vi "Test Copy from Pixmap ARGB.vi"(8 "error in (no error)":errorcluster, 11 "Test Case In":refnum<class "Image.lvclass">) -> (0 "error out":errorcluster, 3 "Test Case Out":refnum<class "Image.lvclass">)   [LabVIEW 2020, in "test.lvlib" / "Image.lvclass"]
uses:
  Image.lvclass
  C:/Program Files (x86)/National Instruments/LabVIEW 2020/vi.lib/Astemes/LUnit/Test Case.lvclass
  <vilib>/picture/picture.llb/imagedata.ctl
  <vilib>/Astemes/LUnit/Test Case.lvclass/Test Case.ctl
  2c93f62b-78d7-4b59-b27c-14bd701a5d71.vi
  26ba0610-68e5-456e-b31e-3dd4b1a41919.vi
  50a666bd-4679-4783-837b-c667b5268c61.vi
  5112621f-71fb-42da-a54b-011c251ba454.vi
  935961b4-3727-4f5b-bf0e-a61aebcf0dca.vi
  image/New Image (ARGB).vi
  image/New Image (Greyscale).vi
  image/Copy Pixmap to Image (ARGB with Mask Output).vi
  image/Copy Pixmap to Image (ARGB Flatten Mask).vi
  7f5bb767-9dbf-47d9-8f44-5f4901e96d00.vi
  e6d5ae8e-bd70-4c65-a769-b7cfb03e80c7.vi
  d454bffa-6717-48ab-b8d5-b1f03345aa55.vi
  image/New Image (ARGB).vi/3321fa97-f432-4e1e-8db9-a0df79aed21b.vi
  image/ARGB Colour to U32 Pixel Value.vi
  image/New Image (Greyscale).vi/6598b9e0-8a08-46f5-91fd-ca1b87217137.vi
  image/Copy Pixmap to Image (ARGB with Mask Output).vi/a116197e-b340-4968-94fb-08de404a21d3.vi
  image/Copy Pixmap to Image (ARGB Flatten Mask).vi/7d03ccf7-b889-4e8d-9f2a-57831e73dbde.vi
  <vilib>/Astemes/LUnit/Append Pass Result.vi
  <vilib>/Astemes/LUnit/Append Fail Result.vi
  <vilib>/Astemes/LUnit/Describe Comparison.vi
  7f5bb767-9dbf-47d9-8f44-5f4901e96d00.vi/9c5d11cd-9439-4240-a1ee-d9baace9c924.vi
  e6d5ae8e-bd70-4c65-a769-b7cfb03e80c7.vi/9c5d11cd-9439-4240-a1ee-d9baace9c924.vi
  d454bffa-6717-48ab-b8d5-b1f03345aa55.vi/9c5d11cd-9439-4240-a1ee-d9baace9c924.vi
  image/FixPixmap.vi
  <vilib>/Astemes/LUnit/Run In UI.vi
  image/Default8bitColourMap.vi
  <vilib>/Utility/error.llb/Clear Errors.vi
  common/Module Path.vi
  <vilib>/Utility/error.llb/Error Cluster From Error Code.vi
  <vilib>/Astemes/LUnit/Describe Variant.vi
  image/image.lvlib
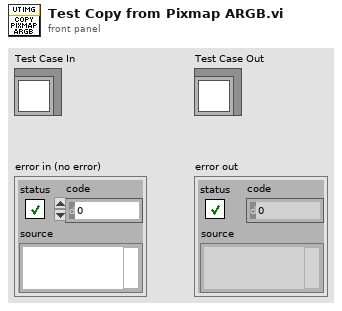
[diagram p1: front panel]
types:
  T1 = enum16{"8 Bit No Mask", "24 Bit No Mask", "32 Bit No Mask", "8 Bit Mask", "24 Bit Mask", "32 Bit Mask", "8 Pixels Wide Masked", "16 Pixels Wide Masked", "8 Bit No Colour Map"}
  T2 = cluster{"left":i16, "top":i16, "right":i16, "bottom":i16}
  T3 = enum16{"8 Bit No Mask", "24 Bit No Mask", "32 Bit No Mask", "8 Bit Mask", "24 Bit Mask", "32 Bit Mask", "8 Pixels Wide Masked", "16 Pixels Wide Masked", "8 Bit No Colour Map"}[]
  T4 = typedef "imagedata.ctl" = cluster{"image type":i32, "image depth":i32, "image":u8[], "mask":u8[], "colors":u32[], "Rectangle":cluster{"left":i16, "top":i16, "right":i16, "bottom":i16}}
  T5 = cluster{"8 No Mask":T4, "8 Mask":T4, "24 No Mask":T4, "24 Mask":T4, "32 No Mask":T4, "32 Mask":T4, "24 Mask - 8 wide":T4, "24 Mask - 16 wide":T4, "8 Bit No Colour Map":T4}
  T6 = typedef "image.lvlib/ARGB Image.ctl" = refnum<data-value>
  T7 = typedef "image.lvlib/Greyscale Image.ctl" = refnum<data-value>
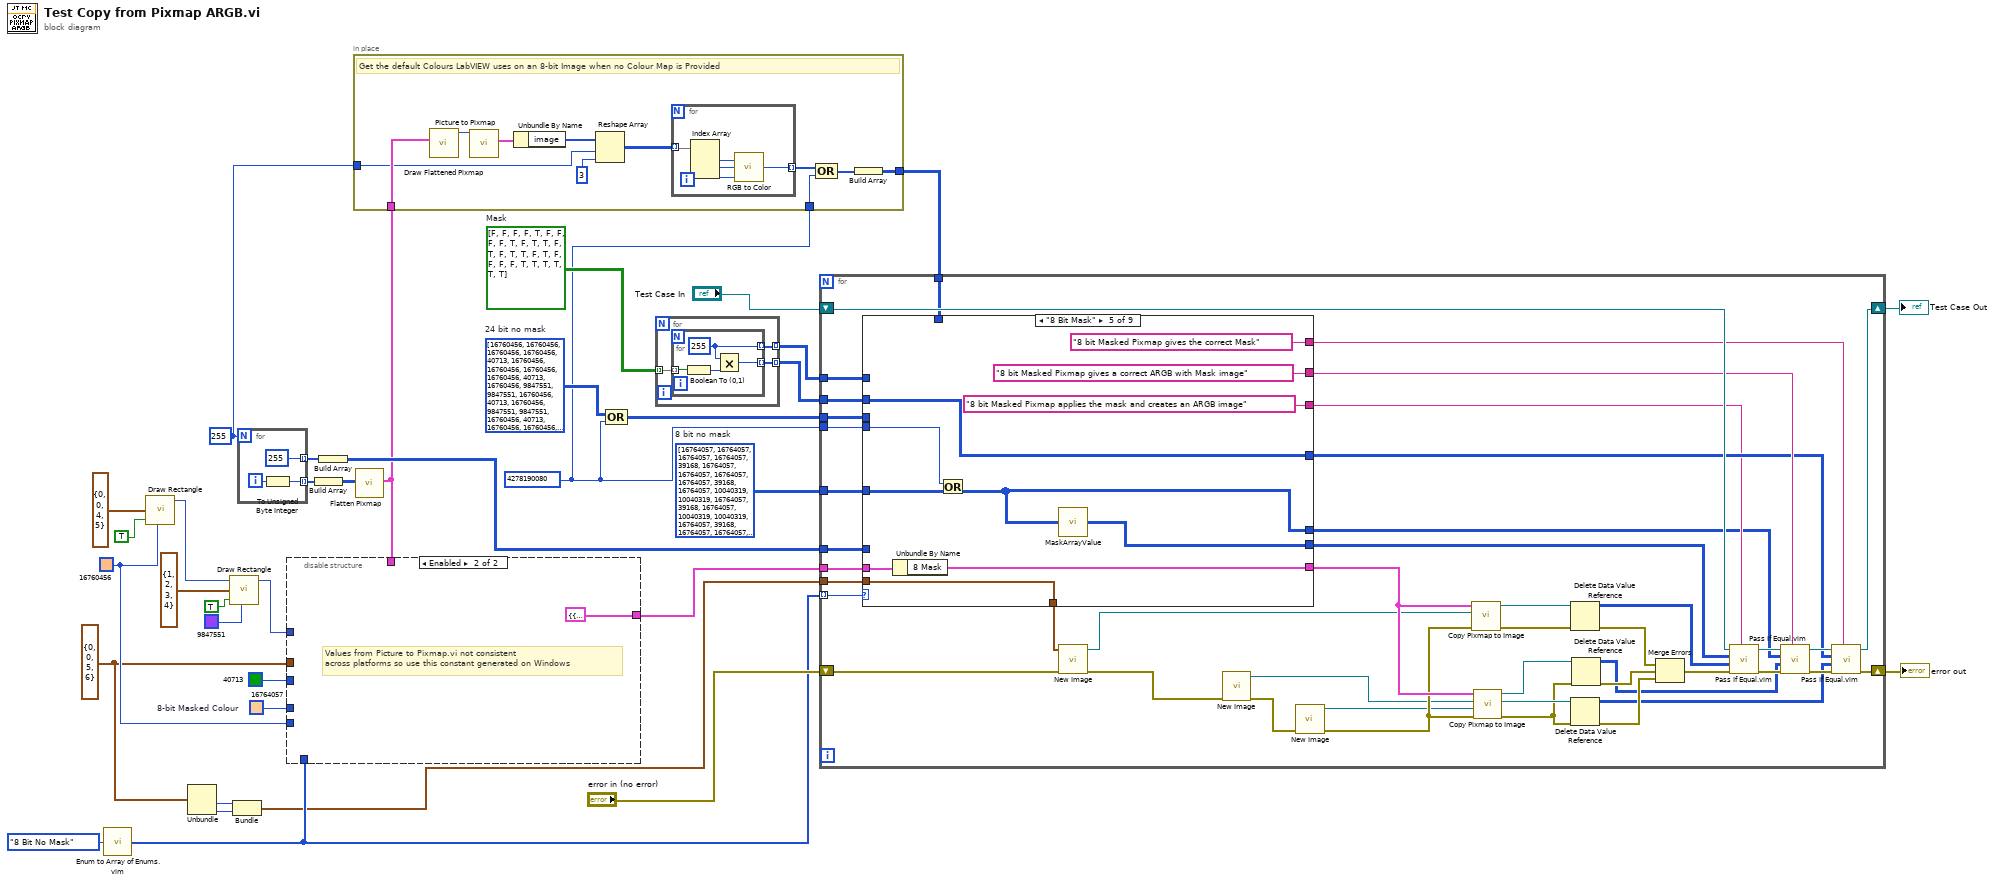
[diagram p0: block diagram]
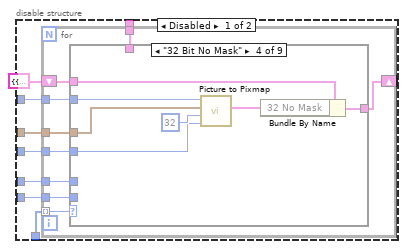
[diagram p2: hidden frame]
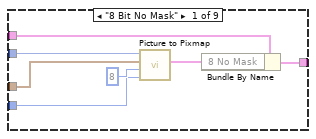
[diagram p3: hidden frame]
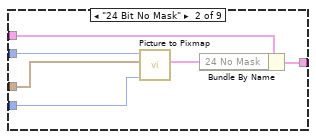
[diagram p4: hidden frame]
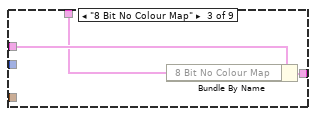
[diagram p5: hidden frame]
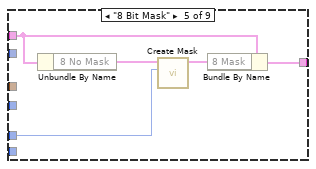
[diagram p6: hidden frame]
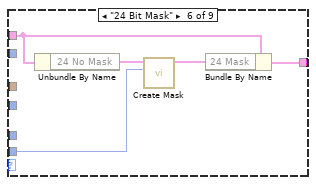
[diagram p7: hidden frame]
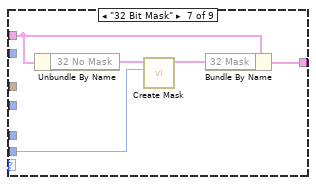
[diagram p8: hidden frame]
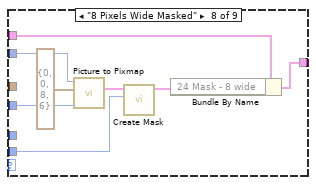
[diagram p9: hidden frame]
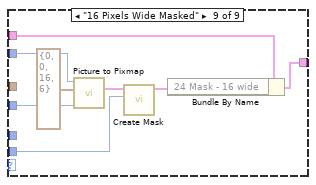
[diagram p10: hidden frame]
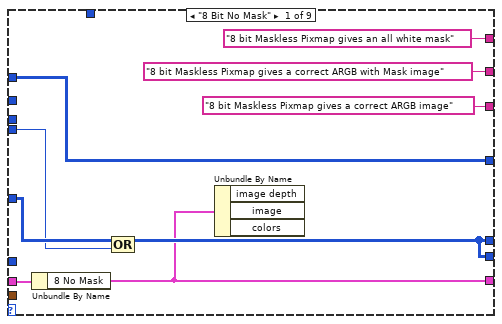
[diagram p11: hidden frame]
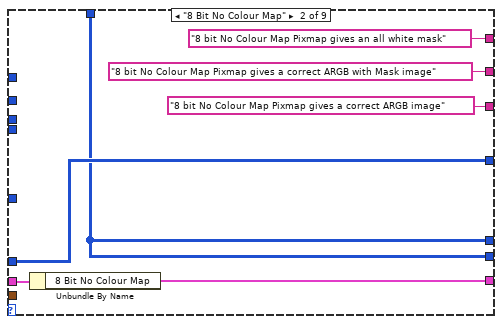
[diagram p12: hidden frame]
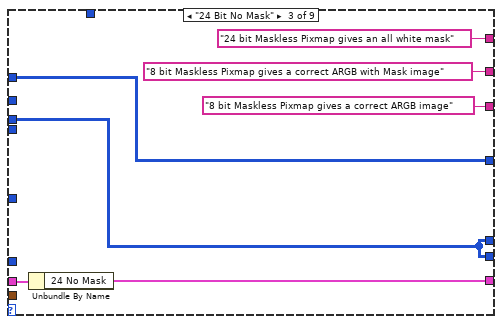
[diagram p13: hidden frame]
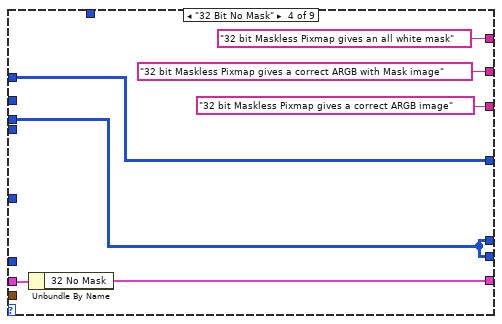
[diagram p14: hidden frame]
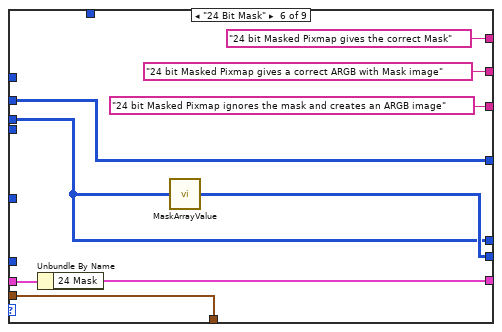
[diagram p15: hidden frame]
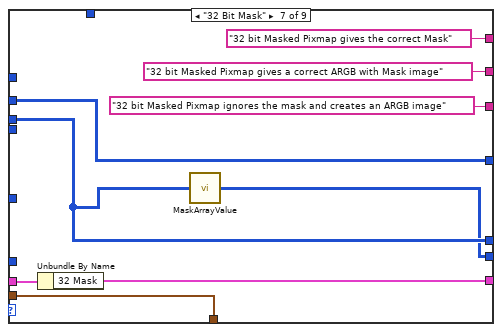
[diagram p16: hidden frame]
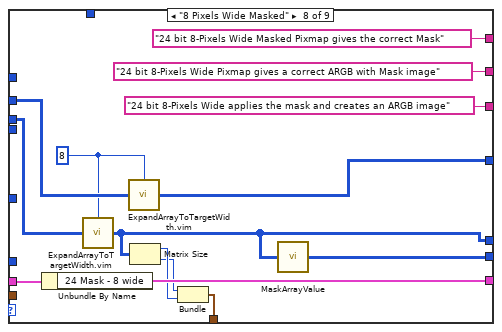
[diagram p17: hidden frame]
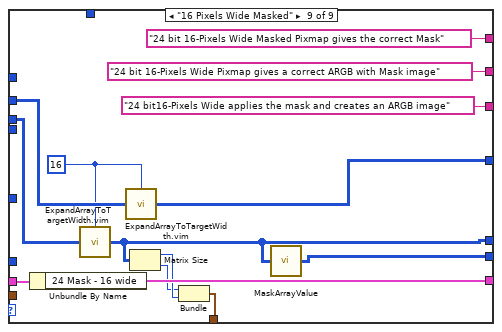
[diagram p18: hidden frame]
diagram:
  w1 = 255
  w9 = u32 16764057  # 8-bit Masked Colour
  w22 = bool[][] [[FALSE, FALSE, FALSE, FALSE, TRUE], [FALSE, FALSE, FALSE, FALSE, TRUE], [FALSE, TRUE, TRUE, FALSE, TRUE], [FALSE, TRUE, TRUE, FALSE, TRUE], [FALSE, FALSE, FALSE, FALSE, TRUE], [TRUE, TRUE, TRUE, TRUE, TRUE]]  # Mask
  w10 = u32[][] [[16764057, 16764057, 16764057, 16764057, 39168], [16764057, 16764057, 16764057, 16764057, 39168], [16764057, 10040319, 10040319, 16764057, 39168], [16764057, 10040319, 10040319, 16764057, 39168], [16764057, 16764057, 16764057, 16764057, 39168], [39168, 39168, 39168, 39168, 39168]]  # 8 bit no mask
  w2 = u32 4278190080
  w25 = u32[][] [[16760456, 16760456, 16760456, 16760456, 40713], [16760456, 16760456, 16760456, 16760456, 40713], [16760456, 9847551, 9847551, 16760456, 40713], [16760456, 9847551, 9847551, 16760456, 40713], [16760456, 16760456, 16760456, 16760456, 40713], [40713, 40713, 40713, 40713, 40713]]  # 24 bit no mask
  w14 = T2 {"left"=0, "top"=0, "right"=5, "bottom"=6} ("rect")
  w17 = u32 16760456 ("color(black)")
  n1 = call "Enum to Array of Enums.vim"("enum"=T1."8 Bit No Mask") -> ("array of enums"=w20:T3)
  n2 = call <vilib>:"Draw Rectangle.vi"("rect"=T2 {"left"=0, "top"=0, "right"=4, "bottom"=5}, "fill?(F)"=TRUE, "color(black)"=w17) -> ("new picture"=w35:picture)  [unwired: 6 in]
  n3 = Unbundle(w14) -> ("right"=w13:i16, "bottom"=w12:i16)  [unwired: 2 out]
  n4 = call <vilib>:"Draw Rectangle.vi"("picture"=w35, "rect"=T2 {"left"=1, "top"=2, "right"=3, "bottom"=4}, "fill?(F)"=TRUE, "color(black)"=u32 9847551) -> ("new picture"=w18:picture)  [unwired: 5 in]
  n5 = Bundle("right"=w13, "bottom"=w12) -> (w11:cluster{"right":i16, "bottom":i16})  [unwired: 1 in]
  n6 = for {
    N: w1 -> [_]
    tunnel: [w37] -> w8 mode=indexing
    tunnel: [u8 255 ("unsigned 8bit integer")] -> w6 mode=indexing
    i -> [w38]
    n7 = To Unsigned Byte Integer(number=w38) -> (unsigned 8bit integer=w37:u8)
  }
  n8 = Build Array(w8) -> (w7:u8[][])
  n9 = Build Array(w6) -> (w5:u8[][])
  n10 = call <vilib>:"Flatten Pixmap.vi"("8-bit pixmap"=w7) -> ("image data"=w4:T4)  [unwired: 10 in]
  n11 = disable-structure shown="Enabled" {
    disable-tunnel: w20 -> [w47 _]
    disable-tunnel: [w45 T5 {"8 No Mask"={"image type"=0, "image depth"=8, "image"=[8, 8, 8, 8, 197, 0, 8, 8, 8, 8, 197, 0, 8, 96, 96, 8, 197, 0, 8, 96, 96, 8, 197, 0, 8, 8, 8, 8, 197, 0, 197, 197, 197, 197, 197, 0], "mask"=[], "colors"=[16777215, 16777164, 16777113, 16777062, 16777011, 16776960, 16764159, 16764108, 16764057, 16764006, 16763955, 16763904, 16751103, 16751052, 16751001, 16750950, 16750899, 16750848, 16738047, 16737996, 16737945, 16737894, 16737843, 16737792, 16724991, 16724940, 16724889, 16724838, 16724787, 16724736, 16711935, 16711884, 16711833, 16711782, 16711731, 16711680, 13434879, 13434828, 13434777, 13434726, 13434675, 13434624, 13421823, 13421772, 13421721, 13421670, 13421619, 13421568, 13408767, 13408716, 13408665, 13408614, 13408563, 13408512, 13395711, 13395660, 13395609, 13395558, 13395507, 13395456, 13382655, 13382604, 13382553, 13382502, 13382451, 13382400, 13369599, 13369548, 13369497, 13369446, 13369395, 13369344, 10092543, 10092492, 10092441, 10092390, 10092339, 10092288, 10079487, 10079436, 10079385, 10079334, 10079283, 10079232, 10066431, 10066380, 10066329, 10066278, 10066227, 10066176, 10053375, 10053324, 10053273, 10053222, 10053171, 10053120, 10040319, 10040268, 10040217, 10040166, 10040115, 10040064, 10027263, 10027212, 10027161, 10027110, 10027059, 10027008, 6750207, 6750156, 6750105, 6750054, 6750003, 6749952, 6737151, 6737100, 6737049, 6736998, 6736947, 6736896, 6724095, 6724044, 6723993, 6723942, 6723891, 6723840, 6711039, 6710988, 6710937, 6710886, 6710835, 6710784, 6697983, 6697932, 6697881, 6697830, 6697779, 6697728, 6684927, 6684876, 6684825, 6684774, 6684723, 6684672, 3407871, 3407820, 3407769, 3407718, 3407667, 3407616, 3394815, 3394764, 3394713, 3394662, 3394611, 3394560, 3381759, 3381708, 3381657, 3381606, 3381555, 3381504, 3368703, 3368652, 3368601, 3368550, 3368499, 3368448, 3355647, 3355596, 3355545, 3355494, 3355443, 3355392, 3342591, 3342540, 3342489, 3342438, 3342387, 3342336, 65535, 65484, 65433, 65382, 65331, 65280, 52479, 52428, 52377, 52326, 52275, 52224, 39423, 39372, 39321, 39270, 39219, 39168, 26367, 26316, 26265, 26214, 26163, 26112, 13311, 13260, 13209, 13158, 13107, 13056, 255, 204, 153, 102, 51, 15597568, 14483456, 12255232, 11141120, 8912896, 7798784, 5570560, 4456448, 2228224, 1114112, 60928, 56576, 47872, 43520, 34816, 30464, 21760, 17408, 8704, 4352, 238, 221, 187, 170, 136, 119, 85, 68, 34, 17, 15658734, 14540253, 12303291, 11184810, 8947848, 7829367, 5592405, 4473924, 2236962, 1118481, 0], "Rectangle"={"left"=0, "top"=0, "right"=5, "bottom"=6}}, "8 Mask"={"image type"=0, "image depth"=8, "image"=[8, 8, 8, 8, 197, 0, 8, 8, 8, 8, 197, 0, 8, 96, 96, 8, 197, 0, 8, 96, 96, 8, 197, 0, 8, 8, 8, 8, 197, 0, 197, 197, 197, 197, 197, 0], "mask"=[15, 255, 15, 255, 111, 255, 111, 255, 15, 255, 255, 255], "colors"=[16777215, 16777164, 16777113, 16777062, 16777011, 16776960, 16764159, 16764108, 16764057, 16764006, 16763955, 16763904, 16751103, 16751052, 16751001, 16750950, 16750899, 16750848, 16738047, 16737996, 16737945, 16737894, 16737843, 16737792, 16724991, 16724940, 16724889, 16724838, 16724787, 16724736, 16711935, 16711884, 16711833, 16711782, 16711731, 16711680, 13434879, 13434828, 13434777, 13434726, 13434675, 13434624, 13421823, 13421772, 13421721, 13421670, 13421619, 13421568, 13408767, 13408716, 13408665, 13408614, 13408563, 13408512, 13395711, 13395660, 13395609, 13395558, 13395507, 13395456, 13382655, 13382604, 13382553, 13382502, 13382451, 13382400, 13369599, 13369548, 13369497, 13369446, 13369395, 13369344, 10092543, 10092492, 10092441, 10092390, 10092339, 10092288, 10079487, 10079436, 10079385, 10079334, 10079283, 10079232, 10066431, 10066380, 10066329, 10066278, 10066227, 10066176, 10053375, 10053324, 10053273, 10053222, 10053171, 10053120, 10040319, 10040268, 10040217, 10040166, 10040115, 10040064, 10027263, 10027212, 10027161, 10027110, 10027059, 10027008, 6750207, 6750156, 6750105, 6750054, 6750003, 6749952, 6737151, 6737100, 6737049, 6736998, 6736947, 6736896, 6724095, 6724044, 6723993, 6723942, 6723891, 6723840, 6711039, 6710988, 6710937, 6710886, 6710835, 6710784, 6697983, 6697932, 6697881, 6697830, 6697779, 6697728, 6684927, 6684876, 6684825, 6684774, 6684723, 6684672, 3407871, 3407820, 3407769, 3407718, 3407667, 3407616, 3394815, 3394764, 3394713, 3394662, 3394611, 3394560, 3381759, 3381708, 3381657, 3381606, 3381555, 3381504, 3368703, 3368652, 3368601, 3368550, 3368499, 3368448, 3355647, 3355596, 3355545, 3355494, 3355443, 3355392, 3342591, 3342540, 3342489, 3342438, 3342387, 3342336, 65535, 65484, 65433, 65382, 65331, 65280, 52479, 52428, 52377, 52326, 52275, 52224, 39423, 39372, 39321, 39270, 39219, 39168, 26367, 26316, 26265, 26214, 26163, 26112, 13311, 13260, 13209, 13158, 13107, 13056, 255, 204, 153, 102, 51, 15597568, 14483456, 12255232, 11141120, 8912896, 7798784, 5570560, 4456448, 2228224, 1114112, 60928, 56576, 47872, 43520, 34816, 30464, 21760, 17408, 8704, 4352, 238, 221, 187, 170, 136, 119, 85, 68, 34, 17, 15658734, 14540253, 12303291, 11184810, 8947848, 7829367, 5592405, 4473924, 2236962, 1118481, 0], "Rectangle"={"left"=0, "top"=0, "right"=5, "bottom"=6}}, "24 No Mask"={"image type"=0, "image depth"=24, "image"=[255, 190, 136, 255, 190, 136, 255, 190, 136, 255, 190, 136, 0, 159, 9, 255, 190, 136, 255, 190, 136, 255, 190, 136, 255, 190, 136, 0, 159, 9, 255, 190, 136, 150, 66, 255, 150, 66, 255, 255, 190, 136, 0, 159, 9, 255, 190, 136, 150, 66, 255, 150, 66, 255, 255, 190, 136, 0, 159, 9, 255, 190, 136, 255, 190, 136, 255, 190, 136, 255, 190, 136, 0, 159, 9, 0, 159, 9, 0, 159, 9, 0, 159, 9, 0, 159, 9, 0, 159, 9], "mask"=[], "colors"=[], "Rectangle"={"left"=0, "top"=0, "right"=5, "bottom"=6}}, "24 Mask"={"image type"=0, "image depth"=24, "image"=[255, 190, 136, 255, 190, 136, 255, 190, 136, 255, 190, 136, 0, 159, 9, 255, 190, 136, 255, 190, 136, 255, 190, 136, 255, 190, 136, 0, 159, 9, 255, 190, 136, 150, 66, 255, 150, 66, 255, 255, 190, 136, 0, 159, 9, 255, 190, 136, 150, 66, 255, 150, 66, 255, 255, 190, 136, 0, 159, 9, 255, 190, 136, 255, 190, 136, 255, 190, 136, 255, 190, 136, 0, 159, 9, 0, 159, 9, 0, 159, 9, 0, 159, 9, 0, 159, 9, 0, 159, 9], "mask"=[15, 255, 15, 255, 111, 255, 111, 255, 15, 255, 255, 255], "colors"=[], "Rectangle"={"left"=0, "top"=0, "right"=5, "bottom"=6}}, "32 No Mask"={"image type"=0, "image depth"=24, "image"=[255, 190, 136, 255, 190, 136, 255, 190, 136, 255, 190, 136, 0, 159, 9, 255, 190, 136, 255, 190, 136, 255, 190, 136, 255, 190, 136, 0, 159, 9, 255, 190, 136, 150, 66, 255, 150, 66, 255, 255, 190, 136, 0, 159, 9, 255, 190, 136, 150, 66, 255, 150, 66, 255, 255, 190, 136, 0, 159, 9, 255, 190, 136, 255, 190, 136, 255, 190, 136, 255, 190, 136, 0, 159, 9, 0, 159, 9, 0, 159, 9, 0, 159, 9, 0, 159, 9, 0, 159, 9], "mask"=[], "colors"=[], "Rectangle"={"left"=0, "top"=0, "right"=5, "bottom"=6}}, "32 Mask"={"image type"=0, "image depth"=24, "image"=[255, 190, 136, 255, 190, 136, 255, 190, 136, 255, 190, 136, 0, 159, 9, 255, 190, 136, 255, 190, 136, 255, 190, 136, 255, 190, 136, 0, 159, 9, 255, 190, 136, 150, 66, 255, 150, 66, 255, 255, 190, 136, 0, 159, 9, 255, 190, 136, 150, 66, 255, 150, 66, 255, 255, 190, 136, 0, 159, 9, 255, 190, 136, 255, 190, 136, 255, 190, 136, 255, 190, 136, 0, 159, 9, 0, 159, 9, 0, 159, 9, 0, 159, 9, 0, 159, 9, 0, 159, 9], "mask"=[15, 255, 15, 255, 111, 255, 111, 255, 15, 255, 255, 255], "colors"=[], "Rectangle"={"left"=0, "top"=0, "right"=5, "bottom"=6}}, "24 Mask - 8 wide"={"image type"=0, "image depth"=24, "image"=[255, 190, 136, 255, 190, 136, 255, 190, 136, 255, 190, 136, 0, 159, 9, 0, 159, 9, 0, 159, 9, 0, 159, 9, 255, 190, 136, 255, 190, 136, 255, 190, 136, 255, 190, 136, 0, 159, 9, 0, 159, 9, 0, 159, 9, 0, 159, 9, 255, 190, 136, 150, 66, 255, 150, 66, 255, 255, 190, 136, 0, 159, 9, 0, 159, 9, 0, 159, 9, 0, 159, 9, 255, 190, 136, 150, 66, 255, 150, 66, 255, 255, 190, 136, 0, 159, 9, 0, 159, 9, 0, 159, 9, 0, 159, 9, 255, 190, 136, 255, 190, 136, 255, 190, 136, 255, 190, 136, 0, 159, 9, 0, 159, 9, 0, 159, 9, 0, 159, 9, 0, 159, 9, 0, 159, 9, 0, 159, 9, 0, 159, 9, 0, 159, 9, 0, 159, 9, 0, 159, 9, 0, 159, 9], "mask"=[15, 255, 15, 255, 111, 255, 111, 255, 15, 255, 255, 255], "colors"=[], "Rectangle"={"left"=0, "top"=0, "right"=8, "bottom"=6}}, "24 Mask - 16 wide"={"image type"=0, "image depth"=24, "image"=[255, 190, 136, 255, 190, 136, 255, 190, 136, 255, 190, 136, 0, 159, 9, 0, 159, 9, 0, 159, 9, 0, 159, 9, 0, 159, 9, 0, 159, 9, 0, 159, 9, 0, 159, 9, 0, 159, 9, 0, 159, 9, 0, 159, 9, 0, 159, 9, 255, 190, 136, 255, 190, 136, 255, 190, 136, 255, 190, 136, 0, 159, 9, 0, 159, 9, 0, 159, 9, 0, 159, 9, 0, 159, 9, 0, 159, 9, 0, 159, 9, 0, 159, 9, 0, 159, 9, 0, 159, 9, 0, 159, 9, 0, 159, 9, 255, 190, 136, 150, 66, 255, 150, 66, 255, 255, 190, 136, 0, 159, 9, 0, 159, 9, 0, 159, 9, 0, 159, 9, 0, 159, 9, 0, 159, 9, 0, 159, 9, 0, 159, 9, 0, 159, 9, 0, 159, 9, 0, 159, 9, 0, 159, 9, 255, 190, 136, 150, 66, 255, 150, 66, 255, 255, 190, 136, 0, 159, 9, 0, 159, 9, 0, 159, 9, 0, 159, 9, 0, 159, 9, 0, 159, 9, 0, 159, 9, 0, 159, 9, 0, 159, 9, 0, 159, 9, 0, 159, 9, 0, 159, 9, 255, 190, 136, 255, 190, 136, 255, 190, 136, 255, 190, 136, 0, 159, 9, 0, 159, 9, 0, 159, 9, 0, 159, 9, 0, 159, 9, 0, 159, 9, 0, 159, 9, 0, 159, 9, 0, 159, 9, 0, 159, 9, 0, 159, 9, 0, 159, 9, 0, 159, 9, 0, 159, 9, 0, 159, 9, 0, 159, 9, 0, 159, 9, 0, 159, 9, 0, 159, 9, 0, 159, 9, 0, 159, 9, 0, 159, 9, 0, 159, 9, 0, 159, 9, 0, 159, 9, 0, 159, 9, 0, 159, 9, 0, 159, 9], "mask"=[15, 255, 15, 255, 111, 255, 111, 255, 15, 255, 255, 255], "colors"=[], "Rectangle"={"left"=0, "top"=0, "right"=16, "bottom"=6}}, "8 Bit No Colour Map"={"image type"=0, "image depth"=8, "image"=[0, 1, 2, 3, 4, 5, 6, 7, 8, 9, 10, 11, 12, 13, 14, 15, 16, 17, 18, 19, 20, 21, 22, 23, 24, 25, 26, 27, 28, 29, 30, 31, 32, 33, 34, 35, 36, 37, 38, 39, 40, 41, 42, 43, 44, 45, 46, 47, 48, 49, 50, 51, 52, 53, 54, 55, 56, 57, 58, 59, 60, 61, 62, 63, 64, 65, 66, 67, 68, 69, 70, 71, 72, 73, 74, 75, 76, 77, 78, 79, 80, 81, 82, 83, 84, 85, 86, 87, 88, 89, 90, 91, 92, 93, 94, 95, 96, 97, 98, 99, 100, 101, 102, 103, 104, 105, 106, 107, 108, 109, 110, 111, 112, 113, 114, 115, 116, 117, 118, 119, 120, 121, 122, 123, 124, 125, 126, 127, 128, 129, 130, 131, 132, 133, 134, 135, 136, 137, 138, 139, 140, 141, 142, 143, 144, 145, 146, 147, 148, 149, 150, 151, 152, 153, 154, 155, 156, 157, 158, 159, 160, 161, 162, 163, 164, 165, 166, 167, 168, 169, 170, 171, 172, 173, 174, 175, 176, 177, 178, 179, 180, 181, 182, 183, 184, 185, 186, 187, 188, 189, 190, 191, 192, 193, 194, 195, 196, 197, 198, 199, 200, 201, 202, 203, 204, 205, 206, 207, 208, 209, 210, 211, 212, 213, 214, 215, 216, 217, 218, 219, 220, 221, 222, 223, 224, 225, 226, 227, 228, 229, 230, 231, 232, 233, 234, 235, 236, 237, 238, 239, 240, 241, 242, 243, 244, 245, 246, 247, 248, 249, 250, 251, 252, 253, 254, 0], "mask"=[], "colors"=[], "Rectangle"={"left"=0, "top"=0, "right"=255, "bottom"=1}}} ("output cluster")] -> w19
    disable-tunnel: w18 -> [w44 _]
    disable-tunnel: w17 -> [w43 _]
    disable-tunnel: u32 40713 ("Background Color") -> [w42 _]
    disable-tunnel: w14 -> [w41 _]
    disable-tunnel: w9 -> [w40 _]
    disable-tunnel: w4 -> [w39 _]
    frame Disabled {
      n12 = for {
        tunnel: w47 -> [w54] mode=indexing
        shift-right: [w55] -> w45
        shift-left: T5 {"8 No Mask"={"image type"=0, "image depth"=0, "image"=[], "mask"=[], "colors"=[], "Rectangle"={"left"=0, "top"=0, "right"=0, "bottom"=0}}, "8 Mask"={"image type"=0, "image depth"=0, "image"=[], "mask"=[], "colors"=[], "Rectangle"={"left"=0, "top"=0, "right"=0, "bottom"=0}}, "24 No Mask"={"image type"=0, "image depth"=0, "image"=[], "mask"=[], "colors"=[], "Rectangle"={"left"=0, "top"=0, "right"=0, "bottom"=0}}, "24 Mask"={"image type"=0, "image depth"=0, "image"=[], "mask"=[], "colors"=[], "Rectangle"={"left"=0, "top"=0, "right"=0, "bottom"=0}}, "32 No Mask"={"image type"=0, "image depth"=0, "image"=[], "mask"=[], "colors"=[], "Rectangle"={"left"=0, "top"=0, "right"=0, "bottom"=0}}, "32 Mask"={"image type"=0, "image depth"=0, "image"=[], "mask"=[], "colors"=[], "Rectangle"={"left"=0, "top"=0, "right"=0, "bottom"=0}}, "24 Mask - 8 wide"={"image type"=0, "image depth"=0, "image"=[], "mask"=[], "colors"=[], "Rectangle"={"left"=0, "top"=0, "right"=0, "bottom"=0}}, "24 Mask - 16 wide"={"image type"=0, "image depth"=0, "image"=[], "mask"=[], "colors"=[], "Rectangle"={"left"=0, "top"=0, "right"=0, "bottom"=0}}, "8 Bit No Colour Map"={"image type"=0, "image depth"=0, "image"=[], "mask"=[], "colors"=[], "Rectangle"={"left"=0, "top"=0, "right"=0, "bottom"=0}}} ("output cluster") -> [w56]
        tunnel: w44 -> [w52]
        tunnel: w41 -> [w53]
        tunnel: w42 -> [w51]
        tunnel: w43 -> [w50]
        tunnel: w40 -> [w49]
        tunnel: w39 -> [w48]
        n13 = case shown="\"32 Bit No Mask\"" w54 {
          tunnel: w56 -> [w63 w69 w72 w79 w83 w88 w93 w102 w110]
          tunnel: [w62 w68 w71 w78 w84 w89 w94 w101 w109] -> w55
          tunnel: w53 -> [w60 w67 _ w76 _ _ _ _ _]
          tunnel: w52 -> [w59 w66 _ w75 _ _ _ w98 w106]
          tunnel: w51 -> [w57 w64 _ w73 _ _ _ w97 w105]
          tunnel: w50 -> [_ _ _ _ _ w85 w90 w95 w103]
          tunnel: w49 -> [_ _ _ _ w80 _ _ _ _]
          tunnel: w48 -> [_ _ w70 _ _ _ _ _ _]
          frame "8 Bit No Mask" {
            n14 = call <vilib>:"Picture to Pixmap.vi"("Background Color"=w57, "depth"=8, "rect"=w60, "picture"=w59) -> ("image data"=w58:T4)  [unwired: 6 in, 1 out]
            n15 = Bundle By Name(cluster=w63, "8 No Mask"=w58) -> (w62:T5)
          }
          frame "24 Bit No Mask" {
            n16 = call <vilib>:"Picture to Pixmap.vi"("Background Color"=w64, "rect"=w67, "picture"=w66) -> ("image data"=w65:T4)  [unwired: 7 in, 1 out]
            n17 = Bundle By Name(cluster=w69, "24 No Mask"=w65) -> (w68:T5)
          }
          frame "8 Bit No Colour Map" {
            n18 = Bundle By Name(cluster=w72, "8 Bit No Colour Map"=w70) -> (w71:T5)
          }
          frame "32 Bit No Mask" {
            n19 = call <vilib>:"Picture to Pixmap.vi"("Background Color"=w73, "depth"=32, "rect"=w76, "picture"=w75) -> ("image data"=w74:T4)  [unwired: 6 in, 1 out]
            n20 = Bundle By Name(cluster=w79, "32 No Mask"=w74) -> (w78:T5)
          }
          frame "8 Bit Mask" {
            n21 = Unbundle By Name(w83) -> ("8 No Mask"=w82:T4)
            n22 = call <vilib>:"Create Mask.vi"("Mask Color (Black)"=w80, "image data"=w82) -> ("image data"=w81:T4)  [unwired: 9 in]
            n23 = Bundle By Name(cluster=w83, "8 Mask"=w81) -> (w84:T5)
          }
          frame "24 Bit Mask" {
            n24 = Unbundle By Name(w88) -> ("24 No Mask"=w87:T4)
            n25 = call <vilib>:"Create Mask.vi"("Mask Color (Black)"=w85, "image data"=w87) -> ("image data"=w86:T4)  [unwired: 9 in]
            n26 = Bundle By Name(cluster=w88, "24 Mask"=w86) -> (w89:T5)
          }
          frame "32 Bit Mask" {
            n27 = Unbundle By Name(w93) -> ("32 No Mask"=w92:T4)
            n28 = call <vilib>:"Create Mask.vi"("Mask Color (Black)"=w90, "image data"=w92) -> ("image data"=w91:T4)  [unwired: 9 in]
            n29 = Bundle By Name(cluster=w93, "32 Mask"=w91) -> (w94:T5)
          }
          frame "8 Pixels Wide Masked" {
            n30 = call <vilib>:"Picture to Pixmap.vi"("Background Color"=w97, "rect"=T2 {"left"=0, "top"=0, "right"=8, "bottom"=6}, "picture"=w98) -> ("image data"=w100:T4)  [unwired: 7 in, 1 out]
            n31 = call <vilib>:"Create Mask.vi"("Mask Color (Black)"=w95, "image data"=w100) -> ("image data"=w99:T4)  [unwired: 9 in]
            n32 = Bundle By Name(cluster=w102, "24 Mask - 8 wide"=w99) -> (w101:T5)
          }
          frame "16 Pixels Wide Masked" {
            n33 = call <vilib>:"Picture to Pixmap.vi"("Background Color"=w105, "rect"=T2 {"left"=0, "top"=0, "right"=16, "bottom"=6}, "picture"=w106) -> ("image data"=w108:T4)  [unwired: 7 in, 1 out]
            n34 = call <vilib>:"Create Mask.vi"("Mask Color (Black)"=w103, "image data"=w108) -> ("image data"=w107:T4)  [unwired: 9 in]
            n35 = Bundle By Name(cluster=w110, "24 Mask - 16 wide"=w107) -> (w109:T5)
          }
        }
      }
    }
    frame Enabled {
      # "Values from Picture to Pixmap.vi not consistent\nacross platforms so use this constant generated on Windows"
    }
  }
  n36 = in-place {
    in-place-border: w4 -> [w122]
    in-place-border: [w118] -> w3
    in-place-border: w2 -> [w115]
    in-place-border: w1 -> [w112]
    # "Get the default Colours LabVIEW uses on an 8-bit Image when no Colour Map is Provided"
    n37 = call <vilib>:"Draw Flattened Pixmap.vi"("image data"=w122) -> ("new picture"=w121:picture)  [unwired: 8 in]
    n38 = call <vilib>:"Picture to Pixmap.vi"("picture"=w121) -> ("image data"=w120:T4)  [unwired: 9 in, 1 out]
    n39 = Unbundle By Name(w120) -> ("image"=w119:u8[])
    n40 = Reshape Array(w119, w112, 3 ("dimension size")) -> (w114:u8[][])
    n41 = for {
      tunnel: w114 -> [w127] mode=indexing
      tunnel: [w123] -> w117 mode=indexing
      n42 = Index Array(array=w127) -> (element #1=w125:u8, element #2=w126:u8, element #3=w124:u8)  [unwired: 3 in]
      n43 = call <vilib>:"RGB to Color.vi"("B"=w124, "G"=w126, "R"=w125) -> ("Color"=w123:u32)
    }
    n44 = Compound Arithmetic op=OR(w117, w115) -> (w116:u32[])
    n45 = Build Array(w116) -> (w118:u32[][])
  }
  n46 = Compound Arithmetic op=OR(w25, w2) -> (w24:u32[][])
  n47 = for "Masks" {
    tunnel: w22 -> [w129] mode=indexing
    tunnel: [w130] -> w23 mode=indexing
    tunnel: [w128] -> w21 mode=indexing
    n48 = for {
      tunnel: [w133] -> w130 mode=indexing
      tunnel: w129 -> [w134] mode=indexing
      tunnel: [w132] -> w128 mode=indexing
      w133 = u8 255 ("unsigned 8bit integer")
      n49 = Boolean To (0,1)(Boolean=w134) -> (0, 1=w131:i16)
      n50 = Multiply(x=w133, y=w131) -> (x*y=w132:u8)
    }
  }
  n51 = for {
    tunnel: w19 -> [w178]
    tunnel: w20 -> [w172] mode=indexing
    shift-right: [w163] -> w26
    shift-left: "error in (no error)" -> [w155]
    shift-right: [w162] -> w29
    shift-left: "Test Case In" -> [w171]
    tunnel: w24 -> [w156]
    tunnel: w10 -> [w159]
    tunnel: w23 -> [w152]
    tunnel: w21 -> [w151]
    tunnel: w11 -> [w146]
    tunnel: w2 -> [w139]
    tunnel: w5 -> [w136]
    tunnel: w3 -> [w135]
    n52 = case shown="\"8 Bit Mask\"" w172 {
      tunnel: w178 -> [w187 w194 w201 w208 w219 w228 w237 w251 w265]
      tunnel: [w179 w193 w200 w207 w218 w227 w236 w250 w264] -> w177
      tunnel: ["8 bit Maskless Pixmap gives an all white mask" ("Description") "8 bit No Colour Map Pixmap gives an all white mask" ("Description") "24 bit Maskless Pixmap gives an all white mask" ("Description") "32 bit Maskless Pixmap gives an all white mask" ("Description") "8 bit Masked Pixmap gives the correct Mask" ("Description") "24 bit Masked Pixmap gives the correct Mask" ("Description") "32 bit Masked Pixmap gives the correct Mask" ("Description") "24 bit 8-Pixels Wide Masked Pixmap gives the correct Mask" ("Description") "24 bit 16-Pixels Wide Masked Pixmap gives the correct Mask" ("Description")] -> w161
      tunnel: ["8 bit Maskless Pixmap gives a correct ARGB with Mask image" ("Description") "8 bit No Colour Map Pixmap gives a correct ARGB with Mask image" ("Description") "8 bit Maskless Pixmap gives a correct ARGB with Mask image" ("Description") "32 bit Maskless Pixmap gives a correct ARGB with Mask image" ("Description") "8 bit Masked Pixmap gives a correct ARGB with Mask image" ("Description") "24 bit Masked Pixmap gives a correct ARGB with Mask image" ("Description") "32 bit Masked Pixmap gives a correct ARGB with Mask image" ("Description") "24 bit 8-Pixels Wide Pixmap gives a correct ARGB with Mask image" ("Description") "24 bit 16-Pixels Wide Pixmap gives a correct ARGB with Mask image" ("Description")] -> w160
      tunnel: [w181 w188 w195 w202 w212 w221 w230 w238 w252] -> w138
      tunnel: w159 -> [w184 _ _ _ w211 _ _ _ _]
      tunnel: [w181 w188 w195 w202 w210 w220 w231 w239 w253] -> w140
      tunnel: [w182 w189 w196 w203 w214 w223 w232 w244 w258] -> w158
      tunnel: ["8 bit Maskless Pixmap gives a correct ARGB image" ("Description") "8 bit No Colour Map Pixmap gives a correct ARGB image" ("Description") "8 bit Maskless Pixmap gives a correct ARGB image" ("Description") "32 bit Maskless Pixmap gives a correct ARGB image" ("Description") "8 bit Masked Pixmap applies the mask and creates an ARGB image" ("Description") "24 bit Masked Pixmap ignores the mask and creates an ARGB image" ("Description") "32 bit Masked Pixmap ignores the mask and creates an ARGB image" ("Description") "24 bit 8-Pixels Wide applies the mask and creates an ARGB image" ("Description") "24 bit16-Pixels Wide applies the mask and creates an ARGB image" ("Description")] -> w157
      tunnel: w156 -> [_ _ w195 w202 _ w220 w231 w246 w260]
      tunnel: w152 -> [w182 _ w196 w203 _ _ _ _ _]
      tunnel: w151 -> [_ _ _ _ w214 w223 w232 w245 w259]
      tunnel: [_ _ _ _ w213 w222 w229 w240 w254] -> w147
      tunnel: w146 -> [_ _ _ _ w213 w222 w229 _ _]
      tunnel: w139 -> [w180 _ _ _ w209 _ _ _ _]
      tunnel: w136 -> [_ w189 _ _ _ _ _ _ _]
      tunnel: w135 -> [_ w188 _ _ _ _ _ _ _]
      frame "8 Bit No Mask" {
        n53 = Unbundle By Name(w187) -> ("8 No Mask"=w179:T4)
        n54 = Compound Arithmetic op=OR(w184, w180) -> (w181:u32[][])
        n55 = Unbundle By Name(w179) -> ()  [unwired: 3 out]
      }
      frame "8 Bit No Colour Map" {
        n56 = Unbundle By Name(w194) -> ("8 Bit No Colour Map"=w193:T4)
      }
      frame "24 Bit No Mask" {
        n57 = Unbundle By Name(w201) -> ("24 No Mask"=w200:T4)
      }
      frame "32 Bit No Mask" {
        n58 = Unbundle By Name(w208) -> ("32 No Mask"=w207:T4)
      }
      frame "8 Bit Mask" {
        n59 = Unbundle By Name(w219) -> ("8 Mask"=w218:T4)
        n60 = Or(x=w209, y=w211) -> (x .or. y?=w210:u32[][])
        n61 = call "MaskArrayValue.vi"("Array In"=w210) -> ("Array out"=w212:u32[][])
      }
      frame "24 Bit Mask" {
        n62 = Unbundle By Name(w228) -> ("24 Mask"=w227:T4)
        n63 = call "MaskArrayValue.vi"("Array In"=w220) -> ("Array out"=w221:u32[][])
      }
      frame "32 Bit Mask" {
        n64 = Unbundle By Name(w237) -> ("32 Mask"=w236:T4)
        n65 = call "MaskArrayValue.vi"("Array In"=w231) -> ("Array out"=w230:u32[][])
      }
      frame "8 Pixels Wide Masked" {
        w243 = 8 ("Target Width")
        n66 = Unbundle By Name(w251) -> ("24 Mask - 8 wide"=w250:T4)
        n67 = call "ExpandArrayToTargetWidth.vim"("Array in"=w246, "Target Width"=w243) -> ("Array out"=w239:u32[][])
        n68 = call "ExpandArrayToTargetWidth.vim"("Array in"=w245, "Target Width"=w243) -> ("Array out"=w244:u8[][])
        n69 = Matrix Size(0:w239) -> (1:w242:i32, 2:w241:i32)
        n70 = Bundle("matrix"=w241, "number of columns"=w242) -> (w240:cluster{"matrix":i32, "number of columns":i32})  [unwired: 1 in]
        n71 = call "MaskArrayValue.vi"("Array In"=w239) -> ("Array out"=w238:u32[][])
      }
      frame "16 Pixels Wide Masked" {
        w257 = 16 ("Target Width")
        n72 = Unbundle By Name(w265) -> ("24 Mask - 16 wide"=w264:T4)
        n73 = call "ExpandArrayToTargetWidth.vim"("Array in"=w260, "Target Width"=w257) -> ("Array out"=w253:u32[][])
        n74 = call "ExpandArrayToTargetWidth.vim"("Array in"=w259, "Target Width"=w257) -> ("Array out"=w258:u8[][])
        n75 = Matrix Size(0:w253) -> (1:w256:i32, 2:w255:i32)
        n76 = Bundle("matrix"=w255, "number of columns"=w256) -> (w254:cluster{"matrix":i32, "number of columns":i32})  [unwired: 1 in]
        n77 = call "MaskArrayValue.vi"("Array In"=w253) -> ("Array out"=w252:u32[][])
      }
    }
    n78 = call-poly "New Image.vi"("error in (no error)"=w155, "Preallocated Image Size (Default: 0,0)"=w147) -> ("error out"=w154:errorcluster, "New ARGB Image"=w153:T6)  [unwired: 8 in]
    n79 = call-poly "New Image.vi"("error in (no error)"=w154) -> ("error out"=w150:errorcluster, "New ARGB Image"=w148:T6)  [unwired: 9 in]
    n80 = call-poly "New Image.vi"("error in (no error)"=w150) -> ("error out"=w176:errorcluster, "New Greyscale Image"=w149:T7)  [unwired: 9 in]
    n81 = call-poly "Copy Pixmap to Image.vi"("error in (no error)"=w176, "ARGB Image Destination"=w153, "Pixmap Image Data"=w177) -> ("error out"=w142:errorcluster, "ARGB Image Destination (duplicate)"=w141:T6)  [unwired: 7 in]
    n82 = call-poly "Copy Pixmap to Image.vi"("error in (no error)"=w176, "Greyscale Image Mask"=w149, "ARGB Image Destination"=w148, "Pixmap Image Data"=w177) -> ("error out"=w144:errorcluster, "Greyscale Image Mask (duplicate)"=w145:T7, "ARGB Image Destination (duplicate)"=w143:T6)  [unwired: 5 in]
    n83 = Delete Data Value Reference(data value reference=w141, error in=w142) -> (data value=w137:u32[][], error out=w175:errorcluster)
    n84 = Delete Data Value Reference(data value reference=w145, error in=w144) -> (data value=w165:u8[][], error out=w173:errorcluster)
    n85 = Delete Data Value Reference(data value reference=w143, error in=w144) -> (data value=w166:u32[][], error out=w174:errorcluster)
    n86 = Merge Errors(w175, w174, w173) -> (w164:errorcluster)
    n87 = call "Pass If Equal.vim"("Description"=w157, "error in (no error)"=w164, "Actual"=w137, "Expected"=w138, "LUnit Test Case In"=w171) -> ("error out"=w168:errorcluster, "LUnit Test Case Out"=w170:refnum<class "Image.lvclass">)  [unwired: 5 in]
    n88 = call "Pass If Equal.vim"("Description"=w160, "error in (no error)"=w168, "Actual"=w166, "Expected"=w140, "LUnit Test Case In"=w170) -> ("error out"=w167:errorcluster, "LUnit Test Case Out"=w169:refnum<class "Image.lvclass">)  [unwired: 5 in]
    n89 = call "Pass If Equal.vim"("Description"=w161, "error in (no error)"=w167, "Actual"=w165, "Expected"=w158, "LUnit Test Case In"=w169) -> ("error out"=w163:errorcluster, "LUnit Test Case Out"=w162:refnum<class "Image.lvclass">)  [unwired: 5 in]
  }
  "error out" <- w26
  "Test Case Out" <- w29
